vi "Test Map to VArray of Clusters.vi"(8 "error in":errorcluster) -> (0 "error out":errorcluster, 2 "passed":bool)   [LabVIEW 2020, in "test_openg_array.lvlib"]
uses:
  test_openg_array.lvlib
  <vilib>/addons/_JKI Toolkits/Caraya/classes/Test/Test.lvclass
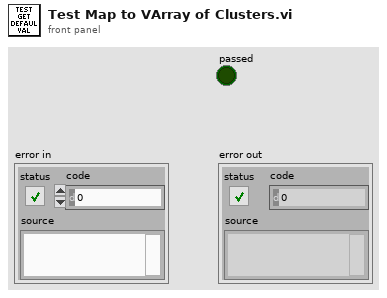
[diagram p1: front panel]
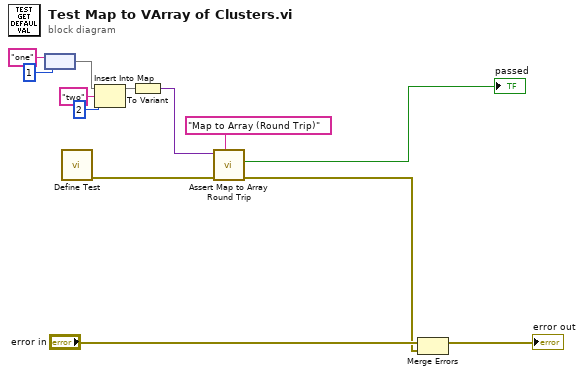
[diagram p0: block diagram]
diagram:
  n1 = node("one" ("key"), 1 ("value")) -> (w10:map{string, i32})
  n2 = call <vilib>:"Define Test.vi"() -> ("error out"=w4:errorcluster)  [unwired: 11 in]
  n3 = Insert Into Map(map in=w10, key="two", value=2) -> (map out=w5:map{string, i32})  [unwired: 2 out]
  n4 = To Variant(anything=w5) -> (Variant=w3:variant)
  n5 = call "Assert Map to Array Round Trip.vi"("Label"="Map to Array (Round Trip)", "error in (no error)"=w4, "Variant"=w3) -> ("error out"=w11:errorcluster, "Passed"=→"passed":bool)  [unwired: 7 in]
  n6 = Merge Errors("error in", w11) -> (→"error out":errorcluster)
